vi "VXM-SetHome.vi"(6 "Set Home All Axes":bool, 8 "error in (no error)":errorcluster, 10 "Subsystem 1, 2, 3":i32, 11 "Message que":T1) -> (0 "error out":errorcluster)   [LabVIEW 2018]
uses:
  Support/MessageQue/MessageQue.ctl
  Support/MessageQue/MessageCluster.ctl
  Support/MessageQue/MessageQue.lvlib
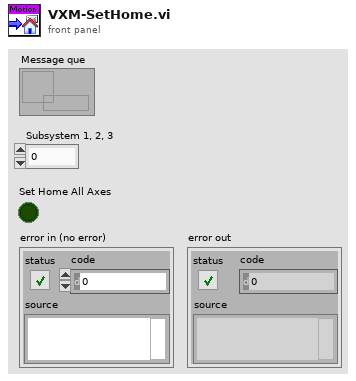
[diagram p1: front panel]
types:
  T1 = typedef "MessageQue.lvlib/MessageQue.ctl" = refnum<queue>
  T2 = cluster{"Subsystem 1, 2, 3":i32, "Set Home All Axes":bool}
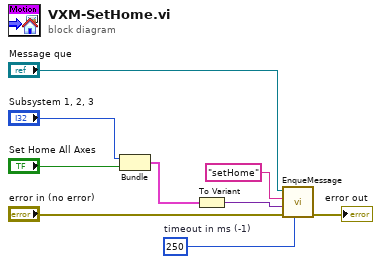
[diagram p0: block diagram]
diagram:
  w8 = 250  # timeout in ms (-1)
  n1 = Bundle("Subsystem 1, 2, 3"="Subsystem 1, 2, 3", "Set Home All Axes"="Set Home All Axes") -> (w2:T2)  [unwired: 1 in]
  n2 = To Variant(anything=w2) -> (Variant=w9:variant)
  n3 = call "EnqueMessage.vi"("timeout in ms (-1)"=w8, "error in"="error in (no error)", "Message Payload"=w9, "Message Command"="setHome", "Message que"="Message que") -> ("error out"=→"error out":errorcluster)  [unwired: 5 in, 1 out]
